vi "Reconstruct_Image.vi"(0 "Data_AI":dbl[](array[numeric])=[1.0, 2.0, 3.0, 4.0, 5.0, 6.0, 7.0, 8.0], 1 "Bidirectionnel?":bool, 5 "Nx":dbl=2.0, 7 "Ny":dbl=2.0, 9 "# Repetition":dbl=2.0, 11 "error in":errorcluster caption="entrée d'erreur") -> (4 "Channel 1":dbl[][](graph), 6 "Data_AI out":dbl[][](array[numeric])=[[1.0, 2.0, 3.0, 4.0, 5.0, 6.0, 7.0, 8.0], [10.0, 20.0, 30.0, 40.0, 50.0, 60.0, 70.0, 80.0]], 15 "error out":errorcluster caption="sortie d'erreur")   [LabVIEW 2026]
uses:
  <vilib>/Analysis/baseanly.llb/Mean (DBL).vi
  <vilib>/Analysis/NI_AALBase.lvlib
panel:
  out "Size OUT":i32[](array[numeric])
  out "Size IN":i32
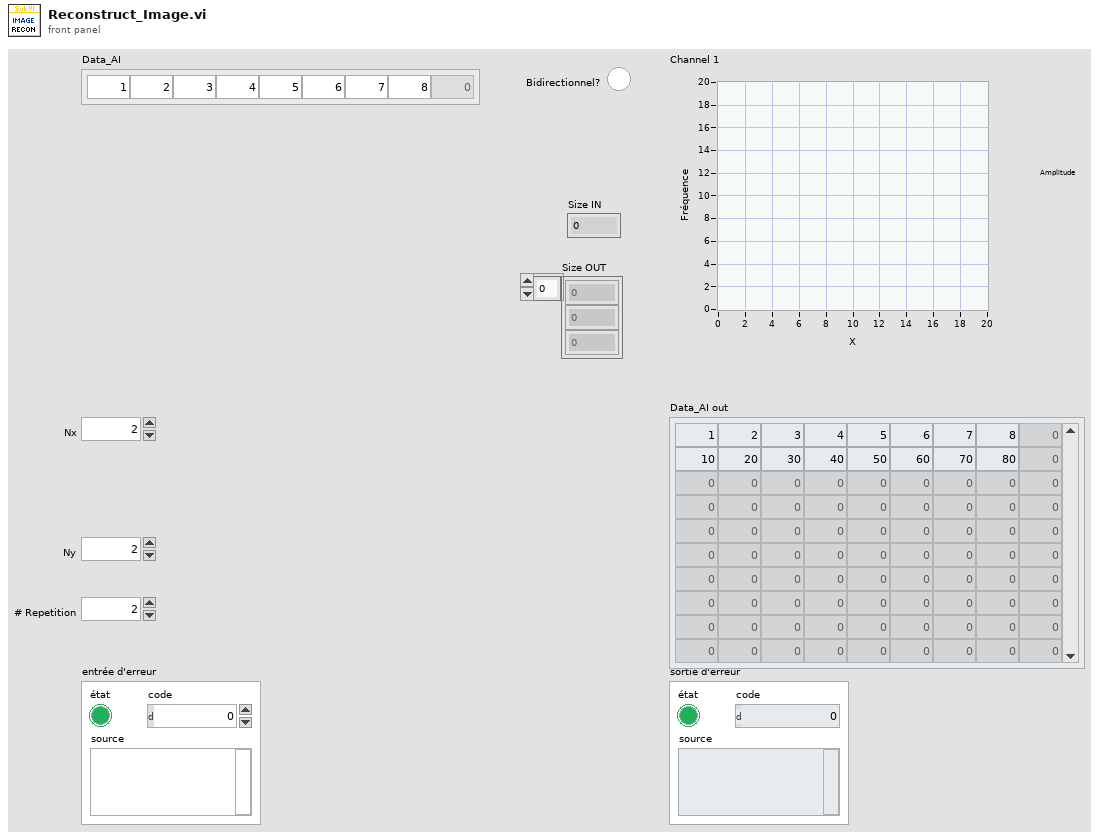
[diagram p1: front panel]
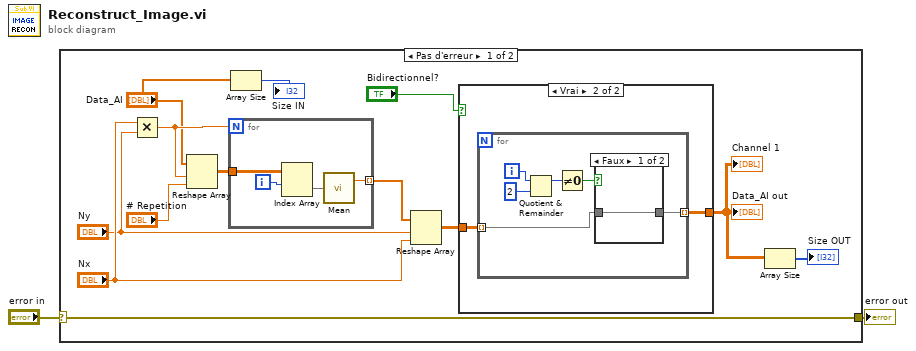
[diagram p0: block diagram]
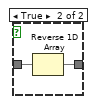
[diagram p3: hidden frame]
diagram:
  n1 = case shown="Pas d'erreur" "error in" {
    selector: "error in" -> [w15 w32]
    tunnel: [w15 w32] -> w1
    frame No Error {
      n2 = Multiply(x="Nx", y="Ny") -> (x*y=w14:dbl)
      n3 = Reshape Array("Data_AI", w14, "# Repetition") -> (w11:dbl[][])
      n4 = for {
        N: w14 -> [_]
        tunnel: w11 -> [w31]
        tunnel: [w28] -> w10 mode=indexing
        i -> [w30]
        n5 = Index Array(array=w31, index (row)=w30) -> (element=w29:dbl[])  [unwired: 1 in]
        n6 = call-poly <vilib>:"Mean.vi"("X"=w29) -> ("mean"=w28:dbl)  [unwired: 1 out]
      }
      n7 = Array Size(array="Data_AI") -> (size(s)=→"Size IN":i32)
      n8 = Reshape Array(w10, "Ny", "Nx") -> (w8:dbl[][])
      n9 = case shown="Vrai" "Bidirectionnel?" {
        tunnel: [w16 w17] -> w4
        tunnel: w8 -> [w16 w18]
        frame False {
        }
        frame True {
          n10 = for {
            tunnel: w18 -> [w20] mode=indexing
            tunnel: [w19] -> w17 mode=indexing
            i -> [w24]
            n11 = Quotient & Remainder(x=w24, y=2) -> (x-y*floor(x/y)=w22:i32)  [unwired: 1 out]
            n12 = Not Equal To 0?(x=w22) -> (x != 0?=w21:bool)
            n13 = case shown="Faux" w21 {
              tunnel: w20 -> [w25 w27]
              tunnel: [w25 w26] -> w19
              frame False {
              }
              frame True {
                n14 = Reverse 1D Array(array=w27) -> (reversed array=w26:dbl[])
              }
            }
          }
        }
      }
      "Channel 1" <- w4
      "Data_AI out" <- w4
      n15 = Array Size(array=w4) -> (size(s)=→"Size OUT":i32[])
    }
    frame Error {
    }
  }
  "error out" <- w1
